vi "Read Units.vi"(8 "error in (no error)":errorcluster, 11 "ElectrometerState in":refnum<class "ElectrometerState.lvclass">) -> (0 "error out":errorcluster, 2 "Units":string[](array[string]), 3 "ElectrometerState out":refnum<class "ElectrometerState.lvclass">)   [LabVIEW 2016]
uses:
  ElectrometerState.lvclass
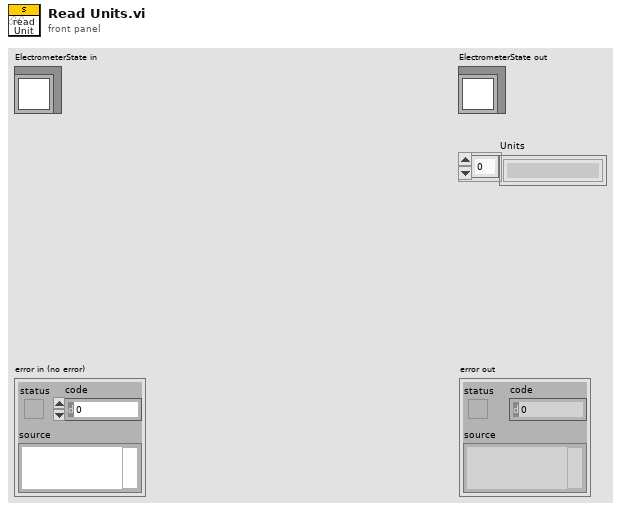
[diagram p1: front panel]
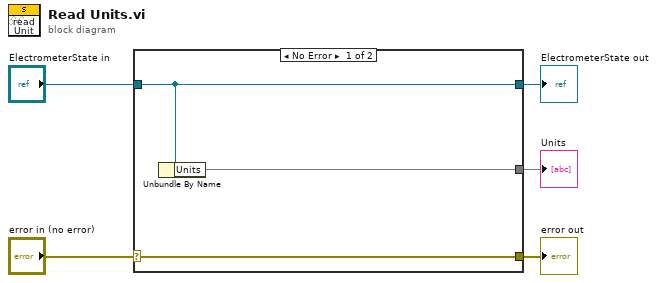
[diagram p0: block diagram]
diagram:
  n1 = case shown="No Error" "error in (no error)" {
    selector: "error in (no error)" -> [w8 w9]
    tunnel: [w8 w9] -> w4
    tunnel: [w7 w10] -> w2
    tunnel: "ElectrometerState in" -> [w7 w10]
    tunnel: [w6 _] -> w1
    frame No Error {
      n2 = Unbundle By Name(w7) -> ("Units"=w6)
    }
    frame Error {
    }
  }
  "error out" <- w4
  "ElectrometerState out" <- w2
  "Units" <- w1
